vi "Discover Local Packages.vi"(8 "error in (no error)":errorcluster, 11 "Artifactory.VIPM in":refnum<class "Artifactory.VIPM.lvclass">) -> (0 "error out":errorcluster, 2 "Local Packages":map{string, string[]}(c390), 3 "Artifactory.VIPM out":refnum<class "Artifactory.VIPM.lvclass">)   [LabVIEW 2021, in "Artifactory.VIPM.lvclass"]
uses:
  Artifactory.VIPM.lvclass
  C:/Repositories/LVOS/Artifactory/lv-src/Artifactory/Artifactory.lvclass
  Artifactory/Artifactory.lvclass/Artifactory.ctl
  Artifactory.VIPM.lvclass/Artifactory.VIPM.ctl
  <vilib>/regexp/Match Regular Expression.xnode
  Artifactory/Artifactory.lvclass
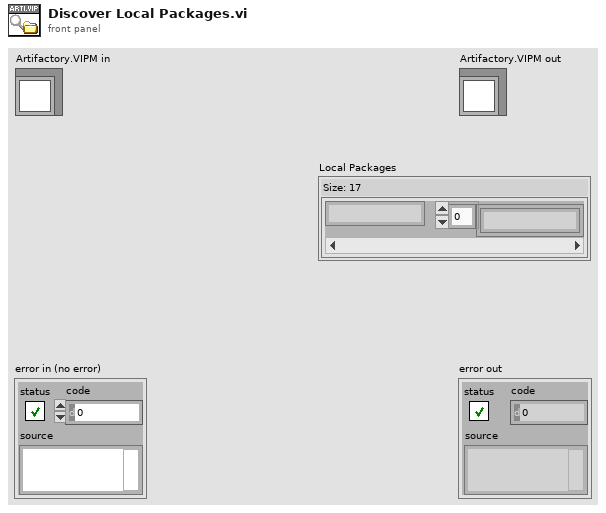
[diagram p1: front panel]
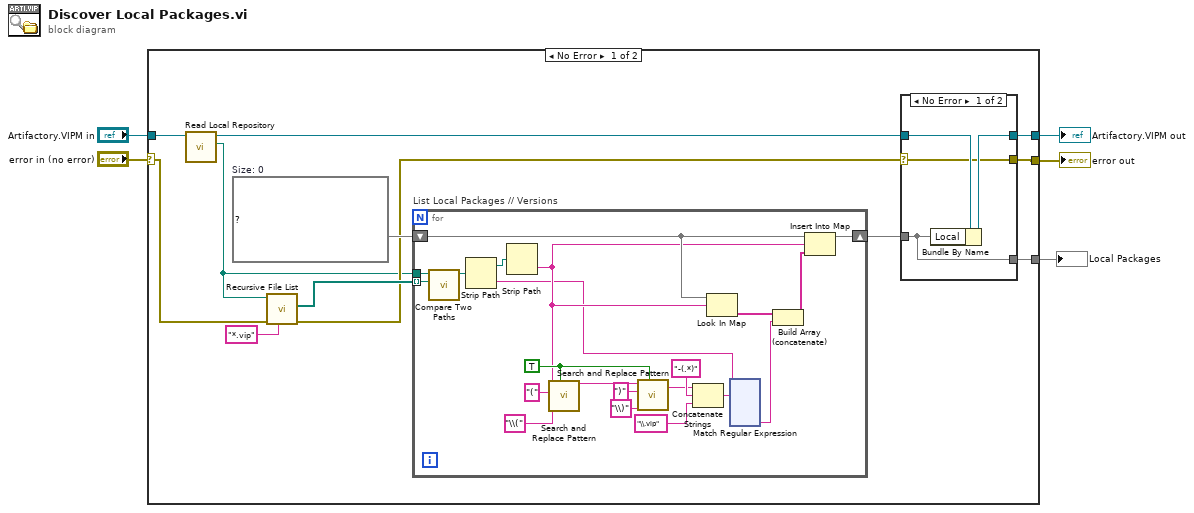
[diagram p0: block diagram]
diagram:
  n1 = case shown="No Error" "error in (no error)" {
    selector: "error in (no error)" -> [w6 w165]
    tunnel: [w16 w165] -> w4
    tunnel: [w17 w164] -> w2
    tunnel: "Artifactory.VIPM in" -> [w8 w164]
    tunnel: [w15 _] -> w1
    frame No Error {
      w12 = map{string, string[]} {}  # Size: 0
      n2 = call "Read Local Repository.vi"("Artifactory in"=w8) -> ("Local Repository"=w7:path, "Artifactory out"=w9:refnum<class "Artifactory.VIPM.lvclass">)  [unwired: 9 in]
      n3 = call <vilib>:"Recursive File List.vi"("pattern"="*.vip", "error in (no error)"=w6, "Folder Path"=w7) -> ("error out"=w10:errorcluster, "All Files in Dir"=w13:path[])  [unwired: 4 in, 3 out]
      n4 = for "List Local Packages // Versions" {
        tunnel: w7 -> [w38]
        tunnel: w13 -> [w37] mode=indexing
        shift-right: [w24] -> w11
        shift-left: w12 -> [w23]
        w32 = TRUE ("replace all? (F)")
        n5 = call <vilib>:"Compare Two Paths.vi"("Path 2"=w37, "Path 1"=w38) -> ("Relative Path from 1 to 2"=w36:path)  [unwired: 6 in, 3 out]
        n6 = Strip Path(path=w36) -> (stripped path=w26:path, name=w18:string)
        n7 = Strip Path(path=w26) -> (name=w22:string)  [unwired: 1 out]
        n8 = call <vilib>:"Search and Replace Pattern.vi"("string"=w22, "regular expression (\"\")"="(" ("regular expression (\"\")"), "replace string (\"\")"="\\(" ("regular expression (\"\")"), "replace all? (F)"=w32) -> ("result string"=w35:string)  [unwired: 1 in, 1 out]
        n9 = call <vilib>:"Search and Replace Pattern.vi"("string"=w35, "regular expression (\"\")"=")" ("regular expression (\"\")"), "replace string (\"\")"="\\)" ("regular expression (\"\")"), "replace all? (F)"=w32) -> ("result string"=w25:string)  [unwired: 1 in, 1 out]
        n10 = Concatenate Strings(w25, "-(.*)" ("string"), "\\.vip" ("regular expression")) -> (w29:string)
        n11 = Look In Map(map=w23, key=w22) -> (value=w21:string[])  [unwired: 1 in, 1 out]
        n12 = xnode "Match Regular Expression"("input string"=w18, "regular expression"=w29) -> ("submatch 1"=w20:string)  [unwired: 4 in, 5 out]
        n13 = Build Array (concatenate)(w21, w20) -> (w19:string[])
        n14 = Insert Into Map(map in=w23, key=w22, value=w19) -> (map out=w24:map{string, string[]})  [unwired: 2 out]
      }
      n15 = case shown="No Error" w10 {
        selector: w10 -> [w159 w162]
        tunnel: w11 -> [w158 _]
        tunnel: w9 -> [w161 w163]
        tunnel: [w160 w163] -> w17
        tunnel: [w159 w162] -> w16
        tunnel: [w158 _] -> w15
        frame No Error {
          n16 = Bundle By Name(cluster=w161, "Local"=w158) -> (w160:refnum<class "Artifactory.VIPM.lvclass">)
        }
        frame Error {
        }
      }
    }
    frame Error {
    }
  }
  "error out" <- w4
  "Artifactory.VIPM out" <- w2
  "Local Packages" <- w1
